vi "Simulationsvariable.vi"() -> ()   [LabVIEW 2019, in "Motor Treiber.lvlib"]
uses:
  Motor Treiber.lvlib
panel:
  out "Direction":bool
  in  "Aktuelle Drehzahl":dbl
  in  "Schrittzeit":timestamp format="%<%x %.3X>T"
  in  "Startzeit":u32
  in  "Soll Drehzahl":dbl
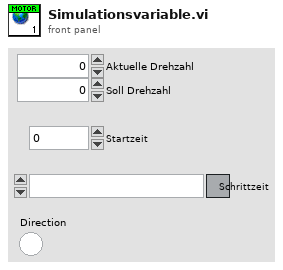
[diagram p1: front panel]
diagram:
